vi "PUMPCONTROL_07 (SubVI).vi"(0 "Port":i32=10, 1 "Pause":bool, 2 "Master start":bool, 3 "shutdown":bool, 8 "Seq in":dbl[][](array[numeric])=[[3.0, 3.0, 7.0], [2.0, 2.0, 2.0], [4.0, 2.0, 100.0]], 23 "reset":bool) -> (4 "Amount now":dbl, 5 "Amount now 2":dbl, 6 "Flow rate out":dbl, 7 "Step amount now":dbl, 9 "Total amount now":dbl, 10 "Total time":dbl, 11 "Numeric 2":i16, 12 "PUMP 1":bool, 13 "Numeric":dbl, 14 "Flow rate":dbl, 15 "Dynamic Data":dynamicdata(waveform), 16 "Target amount":dbl, 17 "Time (min) 2":dbl, 18 "Target amount 2":dbl, 19 "Scale reading":dbl, 20 "Flow rate (g/min)":dbl, 21 "Target (g) 2":dbl, 22 "Target (g)":dbl, 24 "Time (min)":dbl, 25 "Waveform Chart 2":dynamicdata(graph), 26 "Scale weight":dbl, 27 "Amount (g)":dbl)   [LabVIEW 2015]
uses:
  x64/Debug/BERTTA.dll
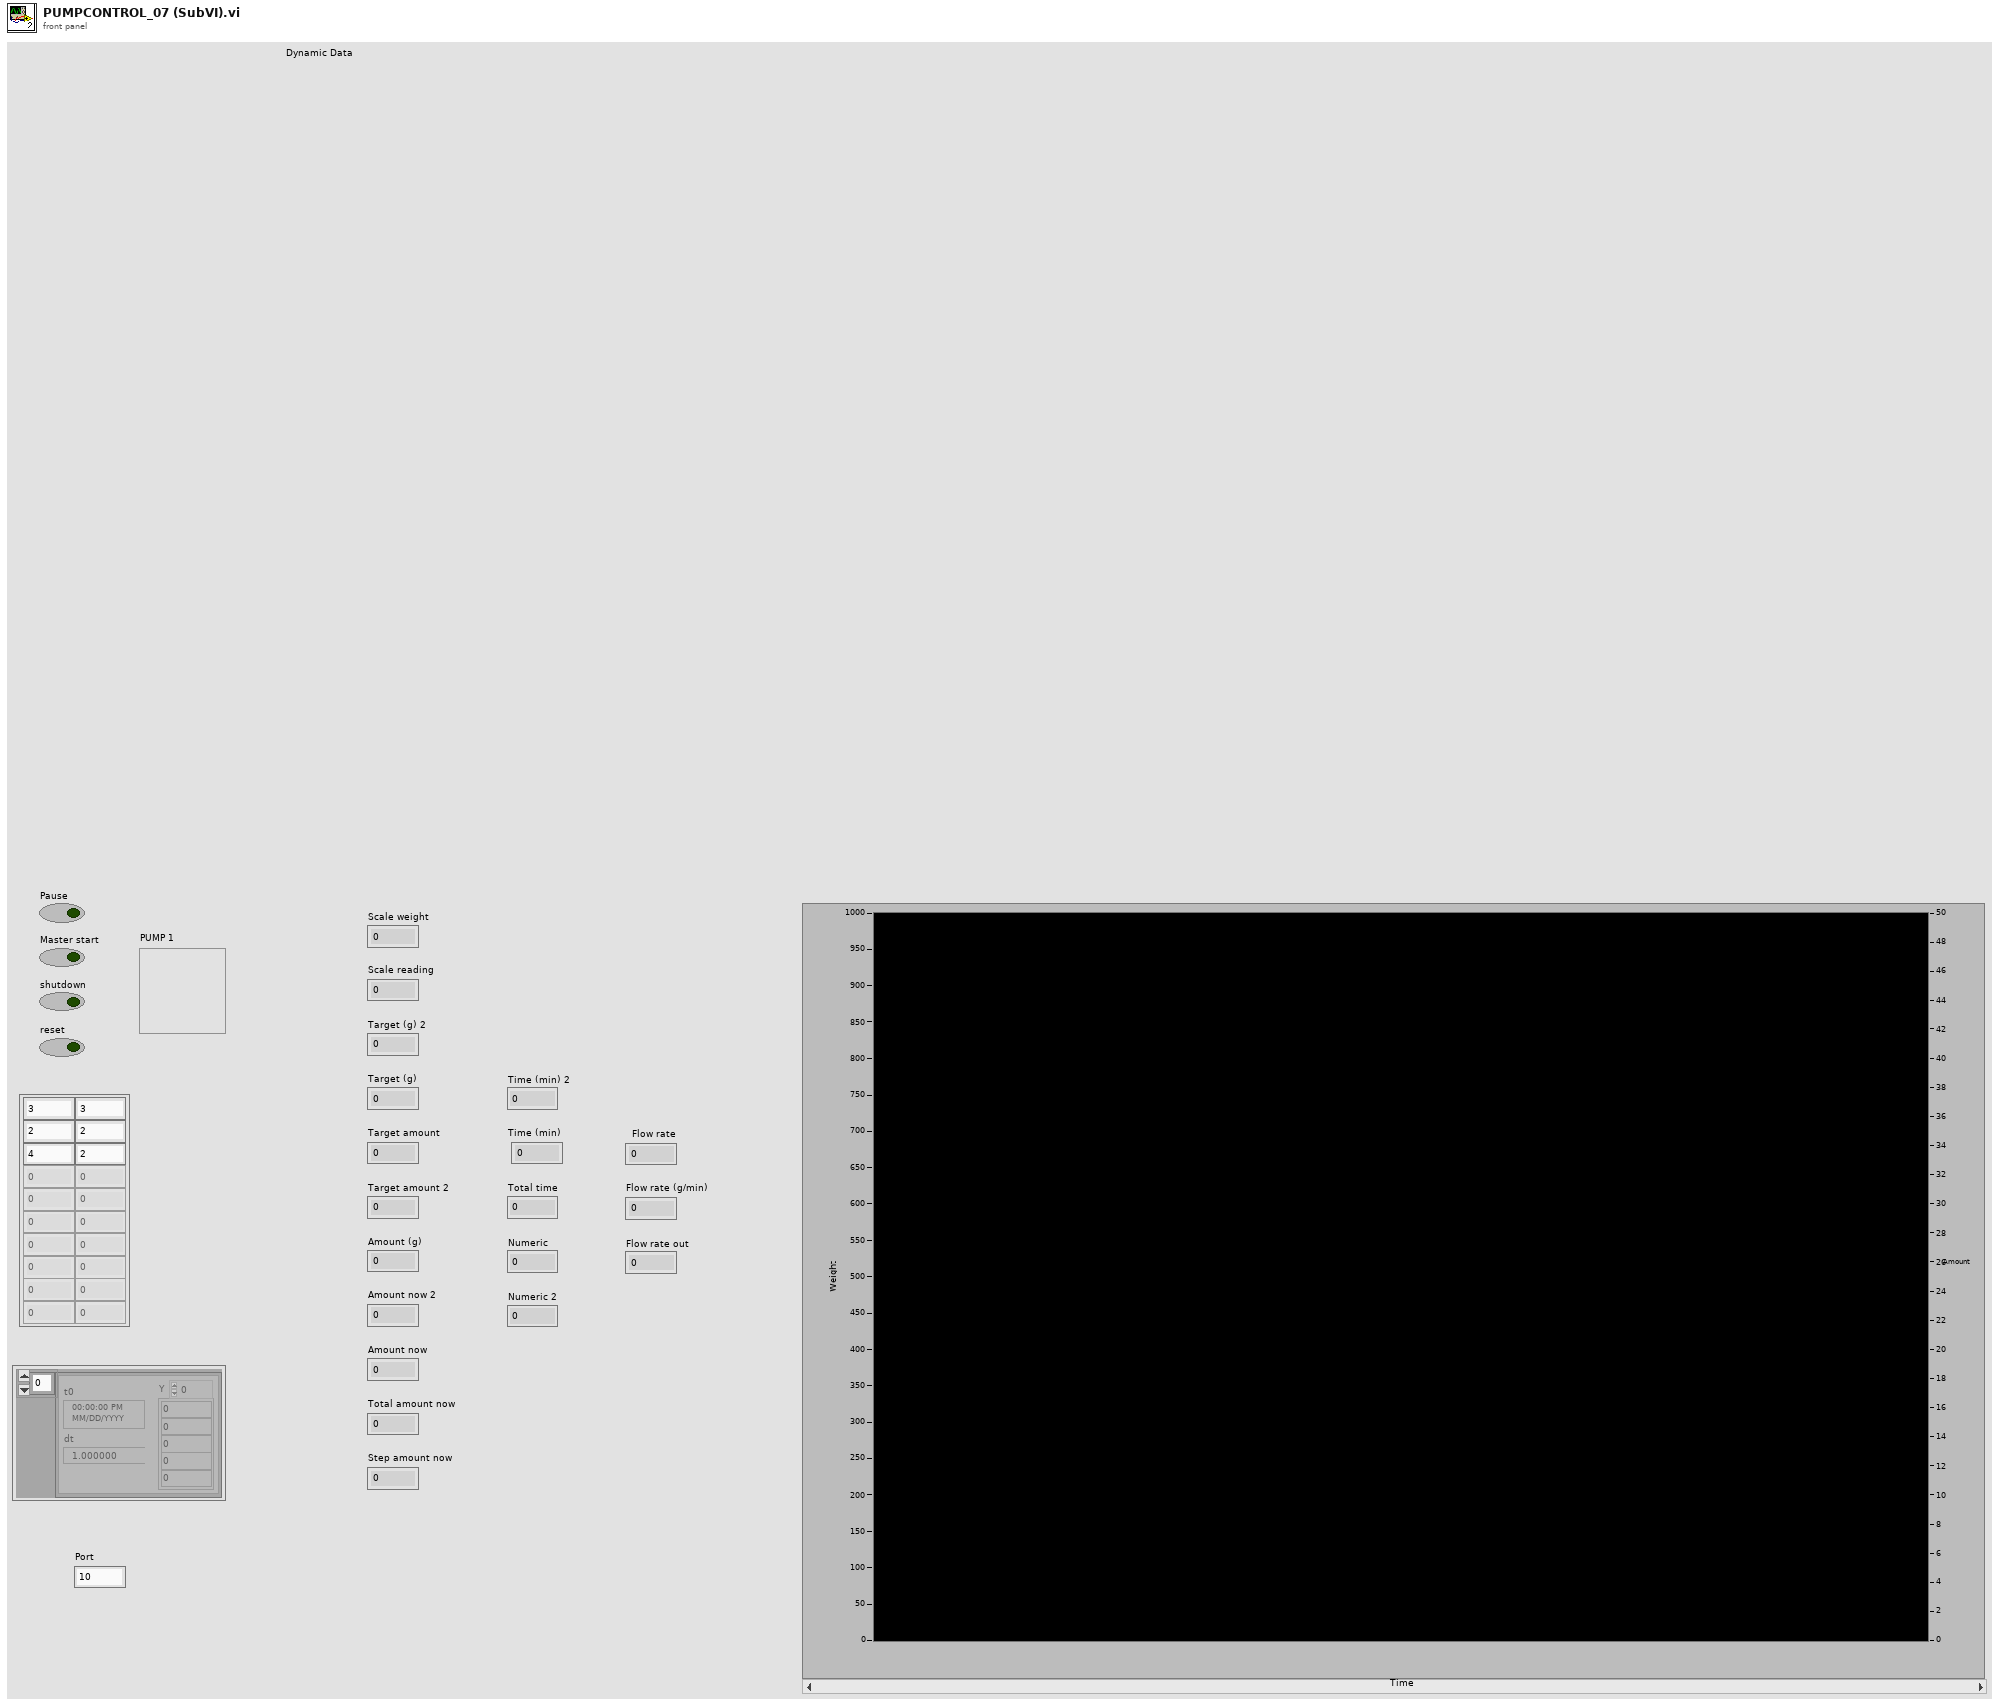
[diagram p1: front panel]
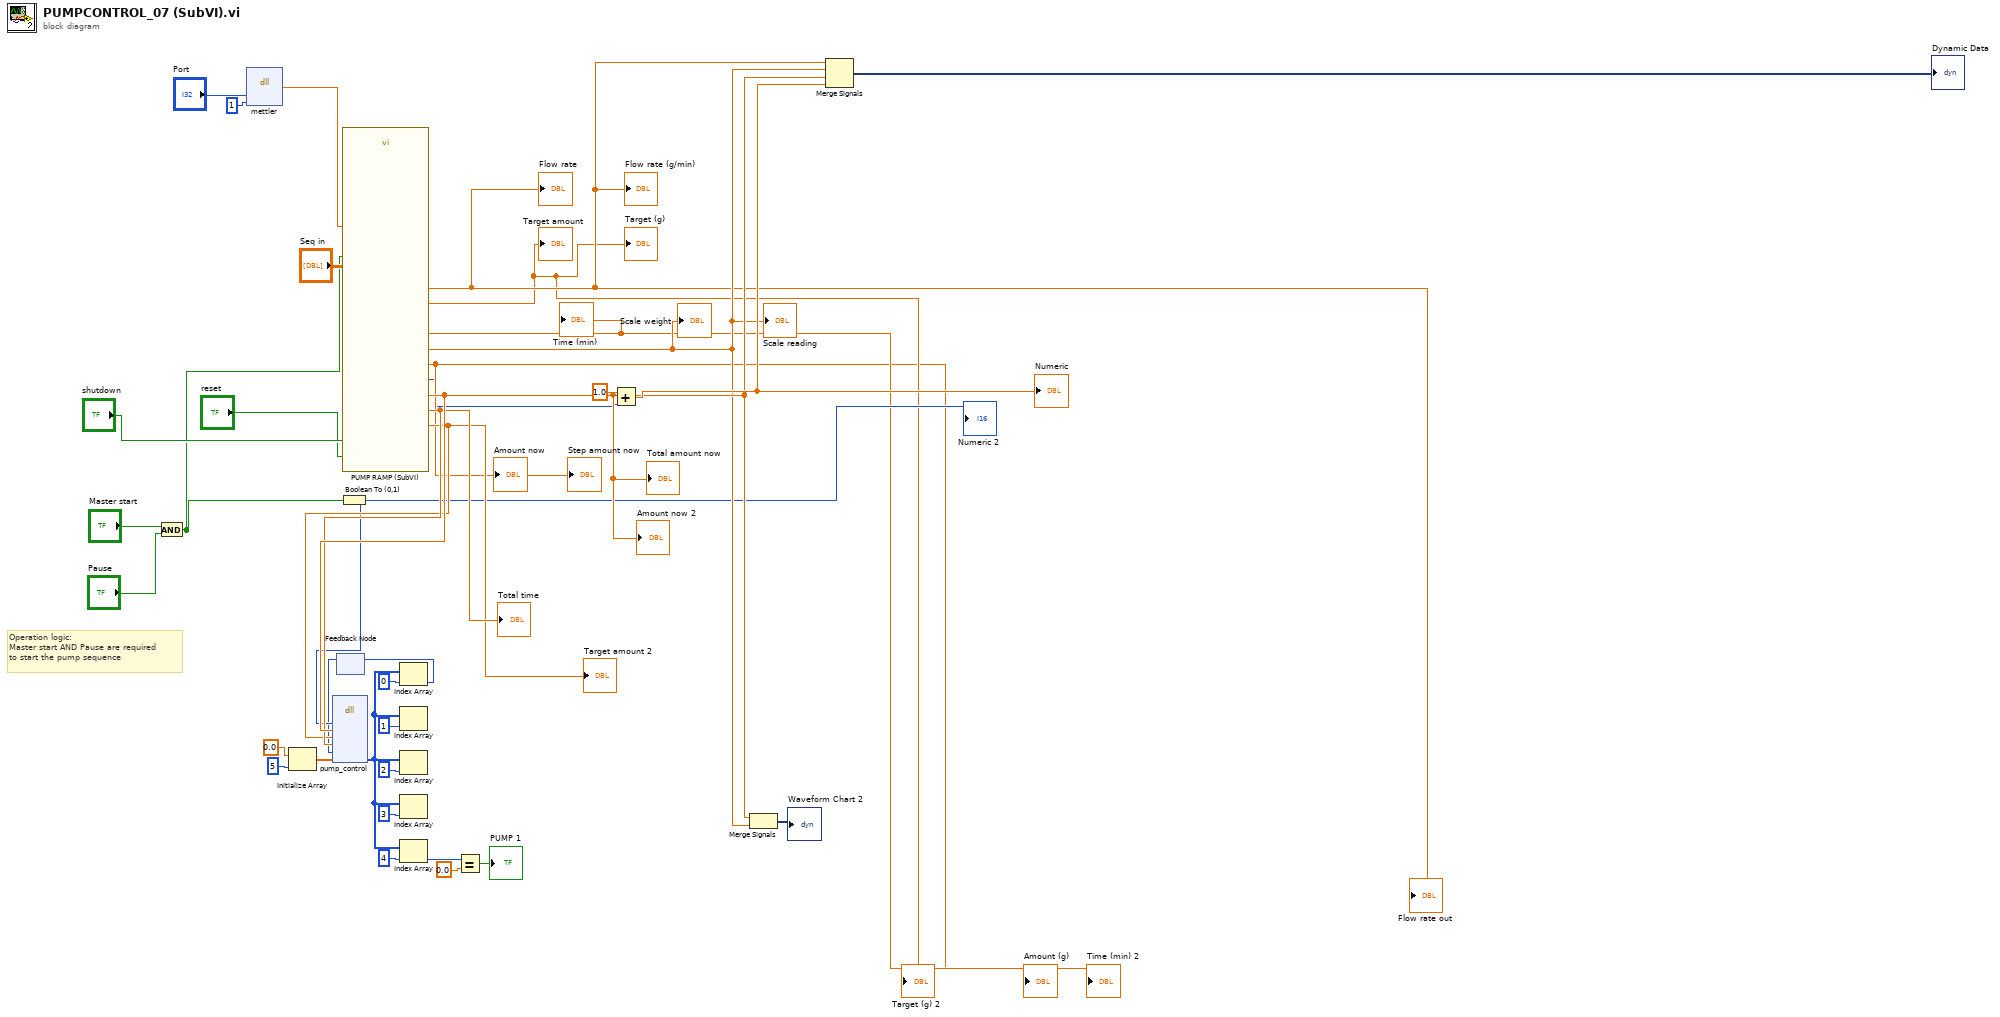
[diagram p0: block diagram]
diagram:
  # "Operation logic:\nMaster start AND Pause are required\nto start the pump sequence"
  n1 = And(x="Master start", y="Pause") -> (x .and. y?=w2:bool)
  n2 = dll-call lib="C:/Users/shresplab/OneDrive - Kemira Oyj/Documents/Visual Studio 2017/Projects/Bertta/BERTTA/x64/Debug/BERTTA.dll" fn="mettler"("port"="Port", "msg"=1) -> ("return type"=w10:dbl)  [unwired: 5 in, 2 out]
  n3 = Initialize Array(0.0 ("element"), 5 ("dimension size")) -> (w13:dbl[])
  n4 = feedback #1() -> (w16:i32)  [unwired: 1 in]
  n5 = Boolean To (0,1)(Boolean=w2) -> (0, 1=w23:i16)
  "Numeric 2" <- w23
  n6 = call "PUMP RAMP (SubVI).vi"("in1"=w10, "Seq in"="Seq in", "Pause"=w2, "Reset"="reset", "shutdown"="shutdown") -> (1:"total amount"=w35:dbl, 2:"total amount"=w29:dbl, "total time"=w30:dbl, "Step"=w6:i32, "Weight"=w34:dbl, "Amount (g)"=→"Step amount now" →"Amount now" →"Amount (g)":dbl, "Time (min)"=→"Time (min)" →"Time (min) 2":dbl, "Target (g)"=→"Target (g)" →"Target amount" →"Target (g) 2":dbl, "Flow rate out"=w33:dbl)  [unwired: 4 in, 2 out]
  "Flow rate (g/min)" <- w33
  "Scale reading" <- w34
  "Scale weight" <- w34
  "Flow rate" <- w33
  "Total amount now" <- w35
  "Total time" <- w30
  "Target amount 2" <- w29
  "Amount now 2" <- w35
  "Flow rate out" <- w33
  n7 = dll-call lib="C:/Users/shresplab/OneDrive - Kemira Oyj/Documents/Visual Studio 2017/Projects/Bertta/BERTTA/x64/Debug/BERTTA.dll" fn="pump_control"("enable"=w23, "amount"=w35, "target"=w29, "time_limit"=w30, "start_time"=w16, "params"=w13) -> ("params"=w25:i32[])  [unwired: 9 in, 2 out]
  n8 = Index Array(array=w25, index=0) -> (element=w15:i32)
  n9 = feedback-in #1(w15) -> ()
  n10 = Index Array(array=w25, index=1) -> ()  [unwired: 1 out]
  n11 = Index Array(array=w25, index=2) -> ()  [unwired: 1 out]
  n12 = Index Array(array=w25, index=3) -> ()  [unwired: 1 out]
  n13 = Index Array(array=w25, index=4) -> (element=w27:i32)
  n14 = Equal?(x=w27, y=0.0) -> (x = y?=→"PUMP 1":bool)
  n15 = Add(x=1.0, y=w6) -> (x+y=w36:dbl)
  "Numeric" <- w36
  n16 = Merge Signals(w35, w34) -> (→"Waveform Chart 2":dynamicdata)
  n17 = Merge Signals(w33, w34, w35, w36) -> (→"Dynamic Data":dynamicdata)
